vi "Arduino LED brightness control.vi"() -> ()   [LabVIEW 2018]
uses:
  <vilib>/Instr/_visa.llb/VISA Configure Serial Port (Instr).vi
panel:
  in  "정지":bool
  in  "둥근 색 상자":u32(colorbox)
  in  "수평 포인터 슬라이드":dbl(slide) scale=0.0..255.0
  in  "port name":refnum<visa-resource-name>
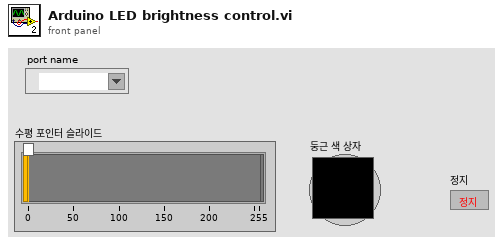
[diagram p1: front panel]
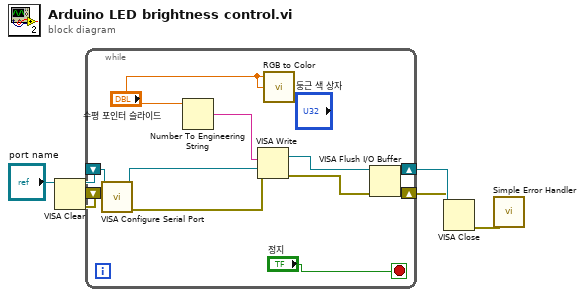
[diagram p0: block diagram]
diagram:
  n1 = VISA Clear(VISA resource name="port name") -> (VISA resource name out=w5:refnum<visa-resource-name>, error out=w6:errorcluster)  [unwired: 1 in]
  n2 = while {
    shift-right: [w10] -> w3
    shift-left: w6 -> [w17]
    shift-right: [w13] -> w4
    shift-left: w5 -> [w16]
    stop <- "정지" stop-if-true
    n3 = call-poly "VISA Configure Serial Port"("VISA resource name"=w16, "error in (no error)"=w17) -> ("VISA resource name out"=w15:refnum<visa-resource-name>, "error out"=w12:errorcluster)  [unwired: 12 in]
    n4 = Number To Engineering String(4:"수평 포인터 슬라이드") -> (0:w9:string)  [unwired: 3 in]
    n5 = VISA Write(VISA resource name=w15, write buffer=w9, error in (no error)=w12) -> (VISA resource name out=w14:refnum<visa-resource-name>, error out=w11:errorcluster)  [unwired: 1 out]
    n6 = call <vilib>:"RGB to Color.vi"("G"="수평 포인터 슬라이드", "R"="수평 포인터 슬라이드") -> ()  [unwired: 1 in, 1 out]
    n7 = VISA Flush I/O Buffer(VISA resource name=w14, error in (no error)=w11) -> (VISA resource name out=w13:refnum<visa-resource-name>, error out=w10:errorcluster)  [unwired: 1 in]
  }
  n8 = VISA Close(VISA resource name=w4, error in (no error)=w3) -> (error out=w1:errorcluster)
  n9 = call <vilib>:"Simple Error Handler.vi"("error in (no error)"=w1) -> ()  [unwired: 4 in, 5 out]
